vi "proptest_instancecount.vi"() -> ()   [LabVIEW 2013, in "NISE_CEF_Tests.lvlib"]
uses:
  Trunk/CEF_TreeControl/serializable configuration/NISE_CEF_serializable configuration.lvclass
  NISE_CEF_Tests.lvlib
panel:
  out "err 538305":errorcluster
  out "no support=ok":bool
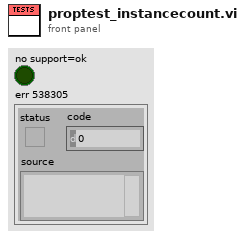
[diagram p1: front panel]
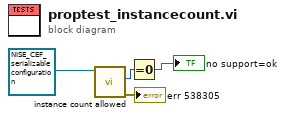
[diagram p0: block diagram]
diagram:
  n1 = call-dynamic "instance count allowed.vi"("configuration in"=refnum<class "NISE_CEF_serializable configuration.lvclass"> refnum ("configuration")) -> ("error out"=→"err 538305":errorcluster, "instances allowed"=w3:i32)  [unwired: 8 in, 1 out]
  n2 = Equal To 0?(x=w3) -> (x = 0?=→"no support=ok":bool)
